vi "Requests.vi"(8 "error in (no error)":errorcluster, 9 "write enable":bool=TRUE, 11 "ICPCON ET-7024 in":refnum<class "ICPCON ET-7024.lvclass">) -> (0 "error out":errorcluster, 3 "ICPCON ET-7024 out":refnum<class "ICPCON ET-7024.lvclass">)   [LabVIEW 2021, in "ICPCON ET-7024.lvclass"]
uses:
  ICPCON ET-7024.lvclass
  D:/my_projects/projects/Algorithms/Labview/21/Modbus/MB_TCP2/MB_TCP.lvclass
  MB_TCP.lvclass/MB_TCP.ctl
  NI_modbus_upd/Ctl/Unit_ID.ctl
  NI_modbus_upd/TCP/TCP.lvclass/TCP.ctl
  NI_modbus_upd/Master Function Definition/Responses/Read Discrete Inputs Response.vi
  NI_modbus_upd/Master network read write.vi
  NI_modbus_upd/Master Function Definition/Requests/Read Discrete Inputs Request.vi
  NI_modbus_upd/Master Function Definition/Responses/Read Coils Response.vi
  NI_modbus_upd/Master Function Definition/Requests/Read Coils Request.vi
  NI_modbus_upd/Master Function Definition/Responses/Read Holding Registers Response.vi
  NI_modbus_upd/Master Function Definition/Requests/Read Holding Registers Request.vi
  NI_modbus_upd/Function data mismatch error1.vi
  NI_modbus_upd/Master Function Definition/Responses/Write Multiple Registers Response.vi
  NI_modbus_upd/Master Function Definition/Requests/Write Multiple Registers Request.vi
  NI_modbus_upd/Master Function Definition/Responses/Write Multiple Coils Response.vi
  NI_modbus_upd/Master Function Definition/Requests/Write Multiple Coils Request.vi
  NI_modbus_upd/Utility/Bytes to Bits1.vi
  NI_modbus_upd/Function code mismatch error1.vi
  NI_modbus_upd/Error Generator1.vi
  NI_modbus_upd/Read ADU Packet Master.vi
  NI_modbus_upd/Write ADU Packet Master.vi
  NI_modbus_upd/Modbus Data Unit (PDU)/Construct PDU1.vi
  NI_modbus_upd/Utility/Bytes to U16s1.vi
  NI_modbus_upd/Utility/U16s to Bytes1.vi
  NI_modbus_upd/Utility/Bits to Bytes1.vi
  NI_modbus_upd/Modbus Data Unit (PDU)/Unflatten to PDU1.vi
  NI_modbus_upd/TCP/Protocol Read.vi
  NI_modbus_upd/TCP/Protocol Write.vi
  <vilib>/Utility/error.llb/Clear Errors.vi
  NI_modbus_upd/Modbus Data Unit (PDU)/Deconstruct PDU1.vi
  NI_modbus_upd/TCP/TCP.lvclass
  ICPCON Registers/ICPCON Registers.lvlib
  MB_TCP.lvclass
  NI_modbus_upd/NI_modbus_upd.lvlib
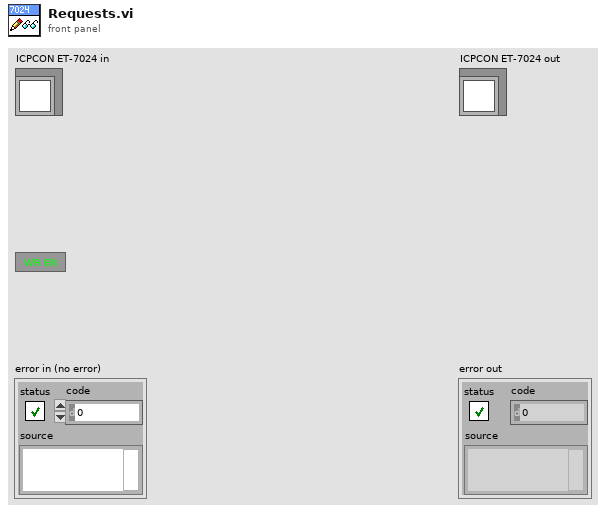
[diagram p1: front panel]
types:
  T1 = typedef "NI_modbus_upd.lvlib/Unit_ID.ctl" = cluster{"Protocol ID":u16, "Unit ID":u8}
  T2 = typedef "ICPCON Registers.lvlib/ICPCON Data.ctl" = cluster{"UTF":refnum<data-value>, "DI":refnum<data-value>, "DW":refnum<data-value>, "DO":refnum<data-value>, "IR":refnum<data-value>, "WR":refnum<data-value>, "OR":refnum<data-value>, "modified":refnum<data-value>}
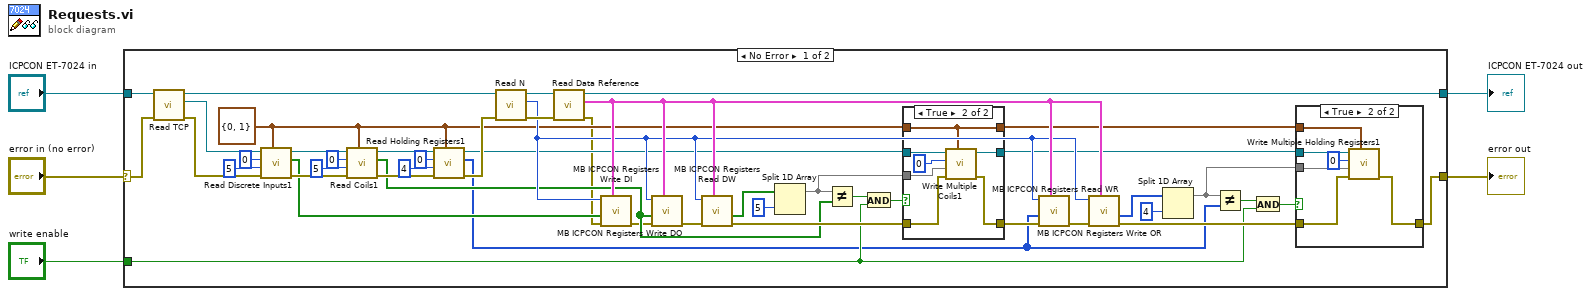
[diagram p0: block diagram]
diagram:
  n1 = case shown="No Error" "error in (no error)" {
    selector: "error in (no error)" -> [w35 w71]
    tunnel: [w26 w71] -> w3
    tunnel: [w33 w70] -> w4
    tunnel: "ICPCON ET-7024 in" -> [w36 w70]
    tunnel: "write enable" -> [w11 _]
    frame No Error {
      w15 = T1 {"Protocol ID"=0, "Unit ID"=1} ("Unit_ID")
      n2 = call "Read TCP.vi"("error in (no error)"=w35, "MB_TCP in"=w36) -> ("error out"=w40:errorcluster, "TCP"=w42:refnum<class "TCP.lvclass">, "MB_TCP out"=w41:refnum<class "ICPCON ET-7024.lvclass">)  [unwired: 7 in]
      n3 = call "Read Discrete Inputs1.vi"("Unit_ID"=w15, "error in (no error)"=w40, "number of discrete inputs"=u16 5, "starting address"=u16 0, "Modbus master in"=w42) -> ("error out"=w43:errorcluster, "discrete input values"=w37:bool[], "Modbus master out"=w39:refnum<class "TCP.lvclass">)  [unwired: 4 in]
      n4 = call "Read Coils1.vi"("Unit_ID"=w15, "error in (no error)"=w43, "number of coils"=u16 5 ("number of discrete inputs"), "starting address"=u16 0, "Modbus master in"=w39) -> ("error out"=w46:errorcluster, "coil values"=w16:bool[], "Modbus master out"=w38:refnum<class "TCP.lvclass">)  [unwired: 4 in]
      n5 = call "Read Holding Registers1.vi"("Unit_ID"=w15, "error in (no error)"=w46, "number of holding registers"=u16 4 ("number of discrete inputs"), "starting address"=u16 0, "Modbus master in"=w38) -> ("error out"=w34:errorcluster, "register values"=w7:u16[], "Modbus master out"=w13:refnum<class "TCP.lvclass">)  [unwired: 4 in]
      n6 = call "Read N.vi"("error in (no error)"=w34, "MB_TCP in"=w41) -> ("error out"=w51:errorcluster, "N"=w17:i32, "MB_TCP out"=w52:refnum<class "ICPCON ET-7024.lvclass">)  [unwired: 7 in]
      n7 = call "Read Data Reference.vi"("error in (no error)"=w51, "MB_TCP in"=w52) -> ("error out"=w6:errorcluster, "Data"=w18:T2, "MB_TCP out"=w33:refnum<class "ICPCON ET-7024.lvclass">)  [unwired: 7 in]
      n8 = call "MB ICPCON Registers Write DI.vi"("Data Reference"=w18, "error in (no error)"=w6, "Bits In"=w37, "N"=w17) -> ("error out"=w10:errorcluster)  [unwired: 7 in]
      n9 = call "MB ICPCON Registers Write DO.vi"("Data Reference"=w18, "error in (no error)"=w10, "Bits In"=w16, "N"=w17) -> ("error out"=w9:errorcluster)  [unwired: 7 in]
      n10 = call "MB ICPCON Registers Read DW.vi"("Data Reference"=w18, "error in (no error)"=w9, "N"=w17) -> ("error out"=w19:errorcluster, "Bits out"=w22:bool[])  [unwired: 7 in]
      n11 = Split 1D Array(array=w22, index=5 ("length")) -> (first subarray=w20:bool[])  [unwired: 1 out]
      n12 = Not Equal?(x=w20, y=w16) -> (x != y?=w24:bool)
      n13 = And(x=w24, y=w11) -> (x .and. y?=w23:bool)
      n14 = case shown="True" w23 {
        tunnel: w19 -> [w55 w61]
        tunnel: [w55 w59] -> w8
        tunnel: w20 -> [_ w62]
        tunnel: w15 -> [w54 w58]
        tunnel: [w54 w58] -> w14
        tunnel: w13 -> [w53 w57]
        tunnel: [w53 w56] -> w12
        frame False {
        }
        frame True {
          n15 = call "Write Multiple Coils1.vi"("Unit_ID"=w58, "error in (no error)"=w61, "coil values"=w62, "starting address"=u16 0, "Modbus master in"=w57) -> ("error out"=w59:errorcluster, "Modbus master out"=w56:refnum<class "TCP.lvclass">)  [unwired: 5 in]
        }
      }
      n16 = call "MB ICPCON Registers Write OR.vi"("Data Reference"=w18, "error in (no error)"=w8, "Words In"=w7, "N"=w17) -> ("error out"=w25:errorcluster)  [unwired: 7 in]
      n17 = call "MB ICPCON Registers Read WR.vi"("Data Reference"=w18, "error in (no error)"=w25, "N"=w17) -> ("error out"=w27:errorcluster, "Words out"=w31:u16[])  [unwired: 7 in]
      n18 = Split 1D Array(array=w31, index=4 ("length")) -> (first subarray=w28:u16[])  [unwired: 1 out]
      n19 = Not Equal?(x=w28, y=w7) -> (x != y?=w30:bool)
      n20 = And(x=w30, y=w11) -> (x .and. y?=w29:bool)
      n21 = case shown="True" w29 {
        tunnel: w27 -> [w63 w68]
        tunnel: [w63 w66] -> w26
        tunnel: w12 -> [_ w69]
        tunnel: w14 -> [_ w64]
        tunnel: w28 -> [_ w65]
        frame False {
        }
        frame True {
          n22 = call "Write Multiple Holding Registers1.vi"("Unit_ID"=w64, "error in (no error)"=w68, "holding register values"=w65, "starting address"=u16 0, "Modbus master in"=w69) -> ("error out"=w66:errorcluster)  [unwired: 5 in, 1 out]
        }
      }
    }
    frame Error {
    }
  }
  "error out" <- w3
  "ICPCON ET-7024 out" <- w4
